vi "ConvertBufferValuesToString.vi"(11 "Buffer Value":T1) -> (3 "Values":string)   [LabVIEW 2012, in "Keithley-2602.lvlib"]
uses:
  Keithley-2602.lvlib
  Public/Controls/BufferValue.ctl
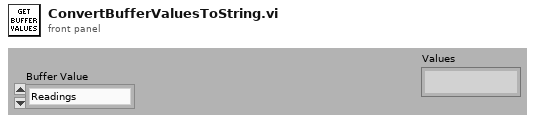
[diagram p1: front panel]
types:
  T1 = typedef "Keithley-2602.lvlib/BufferValue.ctl" = enum16{"Readings", "Source", "Timestamp"}
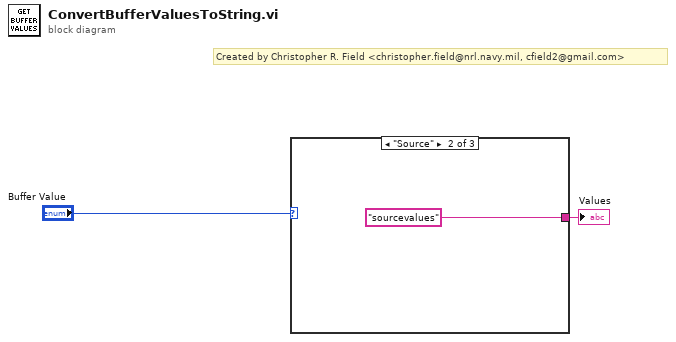
[diagram p0: block diagram]
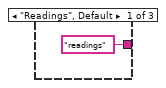
[diagram p2: hidden frame]
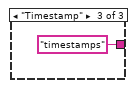
[diagram p3: hidden frame]
diagram:
  # "Created by Christopher R. Field <christopher.field@nrl.navy.mil, cfield2@gmail.com>"
  n1 = case shown="\"Source\"" "Buffer Value" {
    tunnel: ["readings" "sourcevalues" "timestamps"] -> w2
    frame "Readings", Default {
    }
    frame "Source" {
    }
    frame "Timestamp" {
    }
  }
  "Values" <- w2
